vi "storeADCMixedToArray-wang-test2not simplified.vi"(0 "String":string) -> (18 "Graph Data":T1)   [LabVIEW 2014]
uses:
  main/controls/Graph Data.ctl
  <vilib>/Utility/miscctls.llb/LVAnnotationListTypeDef.ctl
  <vilib>/Utility/miscctls.llb/LVCursorListTypeDef.ctl
  main/global/Global ADCarray.vi
panel:
  out "header string":string
  in  "counter 2":i32
  out "Waveform":waveform(dbl)
  out "Graph":waveform(i32)[](graph)
  out "Numeric 2":i32
  out "Numeric":i32
  out "CH7":i32[](array[numeric])
  out "CH6":i32[](array[numeric])
  out "CH5":i32[](array[numeric])
  out "CH4":i32[](array[numeric])
  out "CH3":i32[](array[numeric])
  out "CH2":i32[](array[numeric])
  out "CH1":i32[](array[numeric])
  out "CH0":i32[](array[numeric])
  out "TotalTrigger":i32
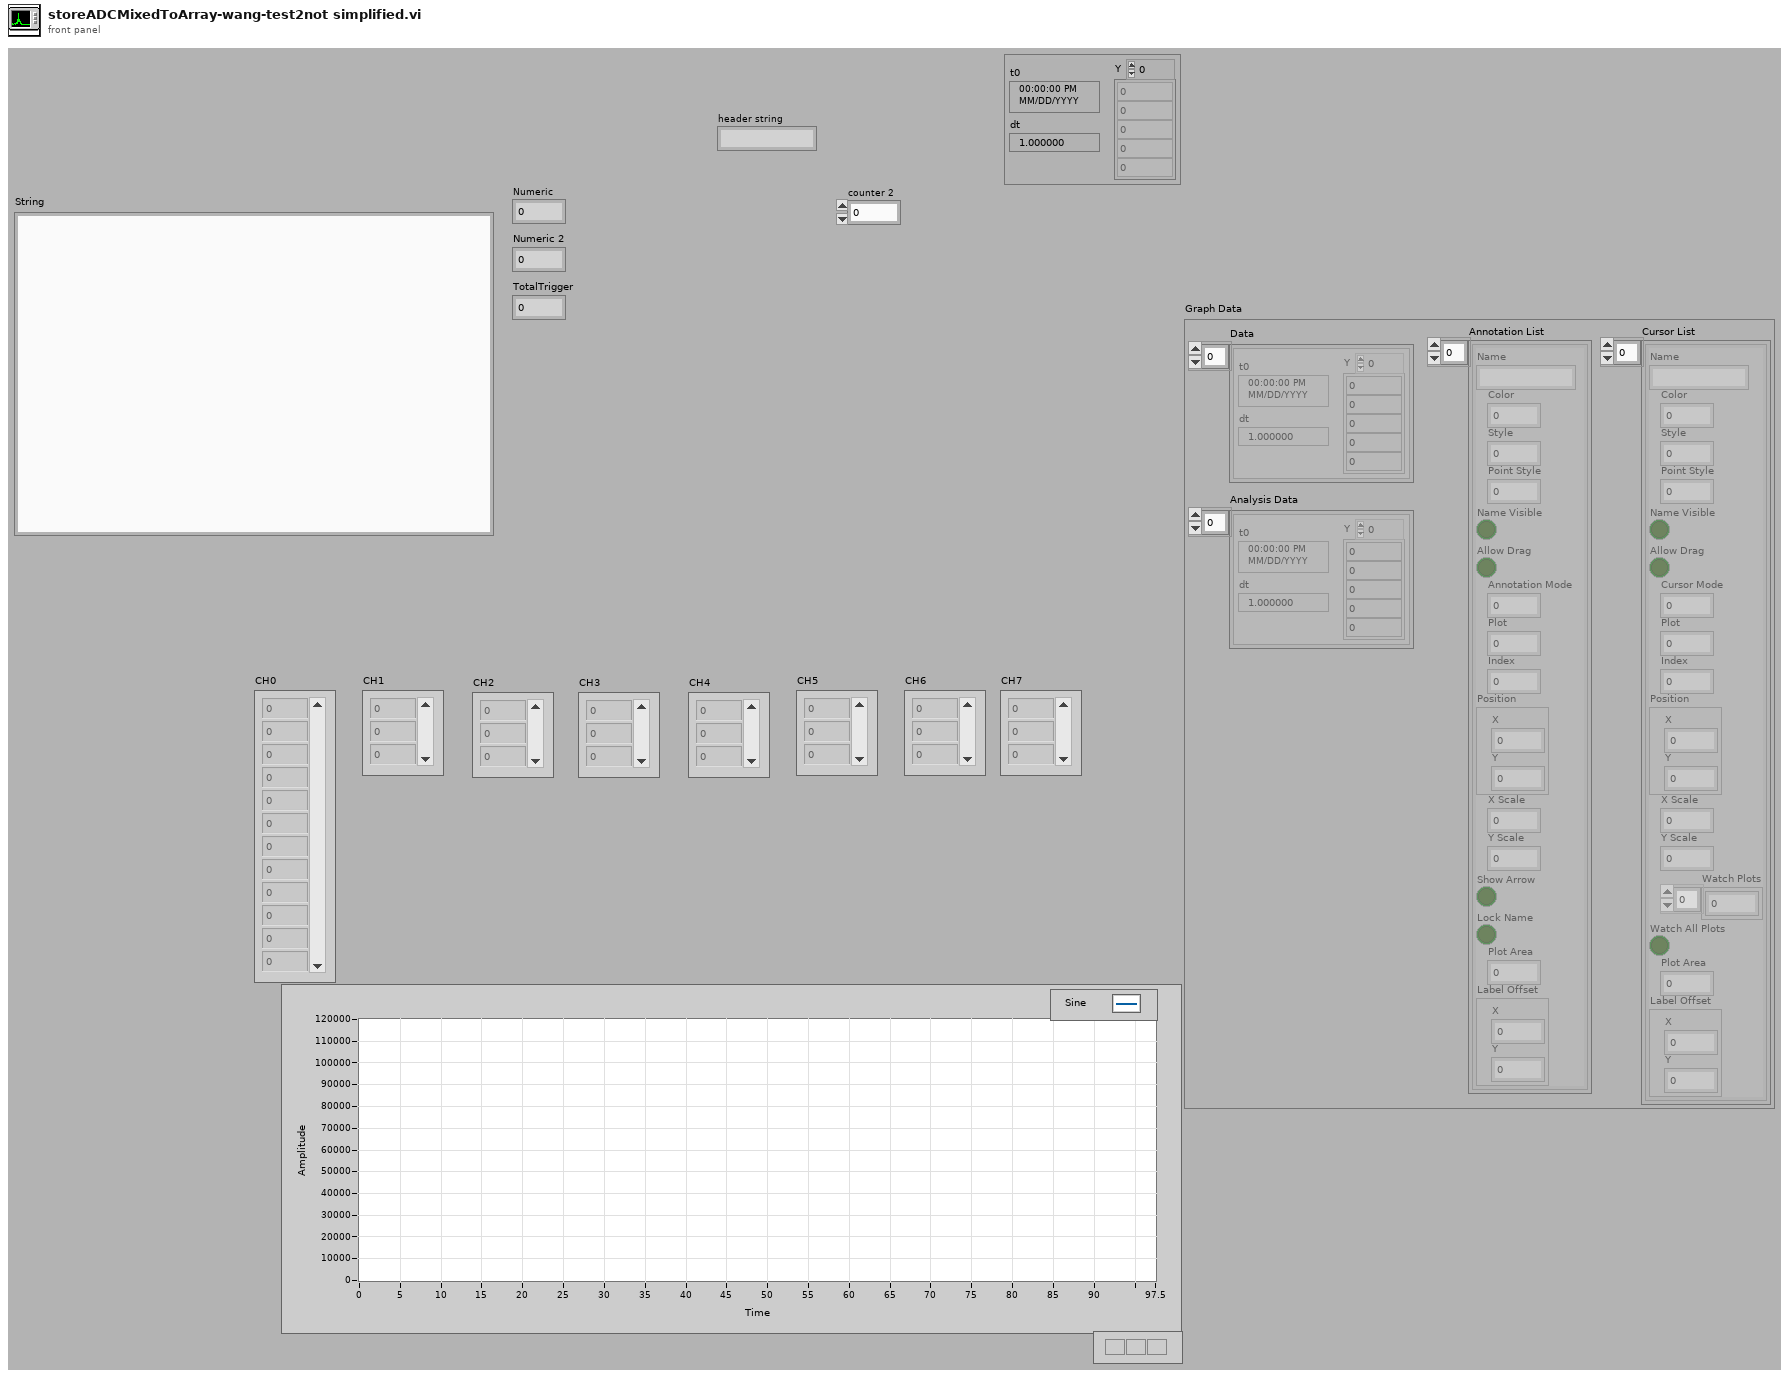
[diagram p1: front panel]
types:
  T1 = typedef "Graph Data.ctl" = cluster{"Data":waveform(dbl)[], "Annotation List":T2, "Cursor List":T3, "Analysis Data":waveform(dbl)[]}
  T2 = typedef "LVAnnotationListTypeDef.ctl" = cluster{"Name":string, "Color":u32, "Style":u8, "Point Style":u8, "Name Visible":bool, "Allow Drag":bool, "Annotation Mode":u32, "Plot":i32, "Index":i32, "Position":cluster{"X":dbl, "Y":dbl}, "X Scale":u32, "Y Scale":u32, "Show Arrow":bool, "Lock Name":bool, "Plot Area":i32, "Label Offset":cluster{"X":dbl, "Y":dbl}}[]
  T3 = typedef "LVCursorListTypeDef.ctl" = cluster{"Name":string, "Color":u32, "Style":u8, "Point Style":u8, "Name Visible":bool, "Allow Drag":bool, "Cursor Mode":u32, "Plot":i32, "Index":i32, "Position":cluster{"X":dbl, "Y":dbl}, "X Scale":u32, "Y Scale":u32, "Watch Plots":i32[], "Watch All Plots":bool, "Plot Area":i32, "Label Offset":cluster{"X":dbl, "Y":dbl}}[]
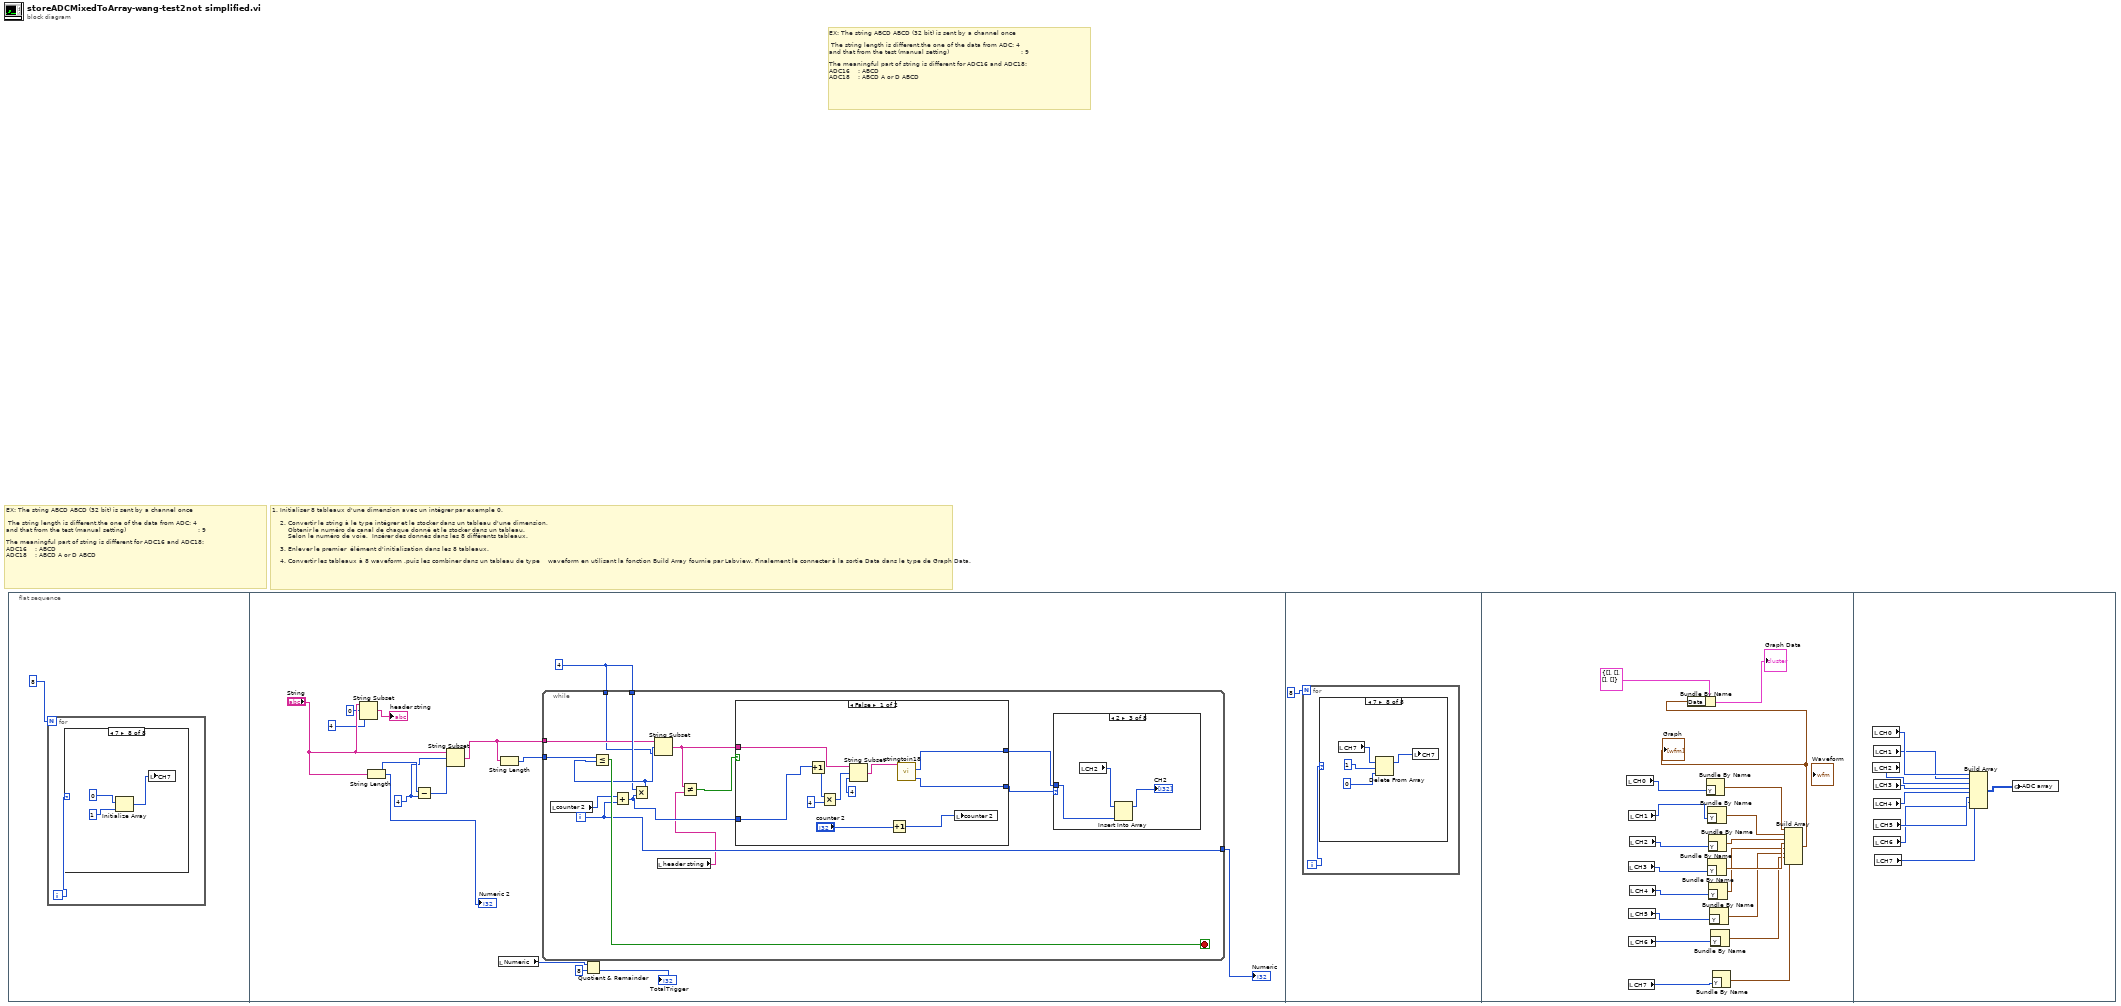
[diagram p0: block diagram]
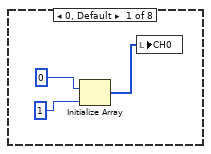
[diagram p2: hidden frame]
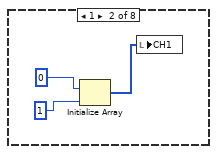
[diagram p3: hidden frame]
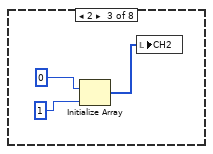
[diagram p4: hidden frame]
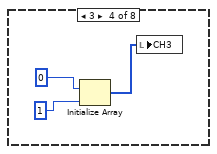
[diagram p5: hidden frame]
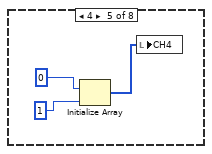
[diagram p6: hidden frame]
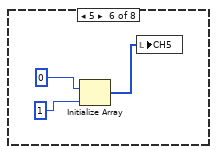
[diagram p7: hidden frame]
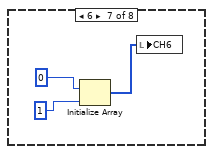
[diagram p8: hidden frame]
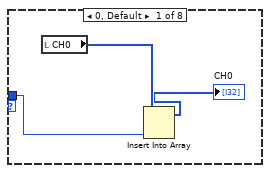
[diagram p9: hidden frame]
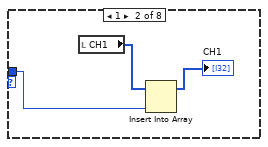
[diagram p10: hidden frame]
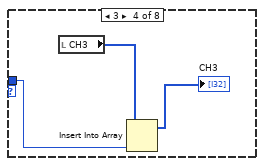
[diagram p11: hidden frame]
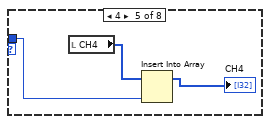
[diagram p12: hidden frame]
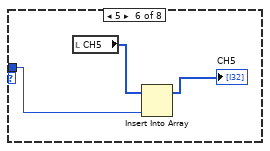
[diagram p13: hidden frame]
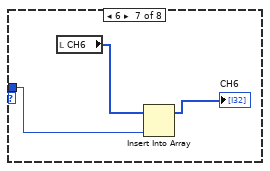
[diagram p14: hidden frame]
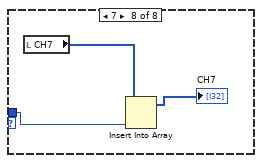
[diagram p15: hidden frame]
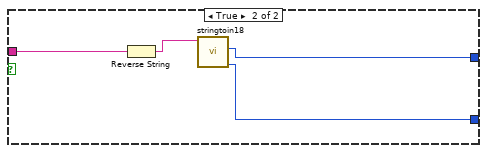
[diagram p16: hidden frame]
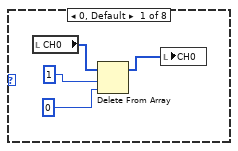
[diagram p17: hidden frame]
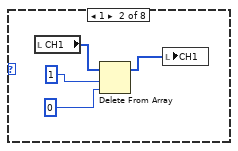
[diagram p18: hidden frame]
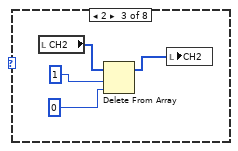
[diagram p19: hidden frame]
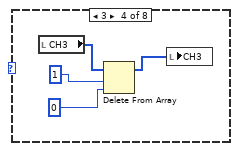
[diagram p20: hidden frame]
diagram:
  # "1. Initialiser 8 tableaux d'une dimension avec un intégrer par exemple 0.\n\n    2.\tConvertir le string à le type intégrer et le stocker dans un tableau d'une dimension,\n        Obtenir le numéro de canal de chaque donné et le stocker dans un tableau.  \n        Selon le numéro de voie,  Insérer des donnés dans les 8 différents tableaux.\n\n    3. Enlever le premier  élément d'initialisation dans les 8 tableaux.\n\n    4. Convertir les tableaux à 8 waveform ,puis les combiner dans un tableau de type    waveform en utilisant la fonction Build Array fournie par Labview. Finalement le connecter à la sortie Data dans le type de Graph Data."
  # "EX: The string ABCD ABCD (32 bit) is sent by a channel once                \n\n The string length is different,the one of the data from ADC: 4\nand that from the test (manual setting)                                    : 9\n\nThe meaningful part of string is different for ADC16 and ADC18:\nADC16    : ABCD                          \nADC18    : ABCD A or D ABCD"
  # "EX: The string ABCD ABCD (32 bit) is sent by a channel once                \n\n The string length is different,the one of the data from ADC: 4\nand that from the test (manual setting)                                    : 9\n\nThe meaningful part of string is different for ADC16 and ADC18:\nADC16    : ABCD                          \nADC18    : ABCD A or D ABCD"
  n1 = flat-sequence {
    frame #0 {
      n2 = for {
        N: 8 -> [_]
        i -> [w2]
        n3 = case shown="7" w2 {
          frame 0, Default {
            n4 = Initialize Array(0, 1) -> (w3:i32[])
            n5 = local write "CH0"(w3) -> ()
          }
          frame 1 {
            n6 = Initialize Array(0, 1) -> (w6:i32[])
            n7 = local write "CH1"(w6) -> ()
          }
          frame 2 {
            n8 = Initialize Array(0, 1) -> (w9:i32[])
            n9 = local write "CH2"(w9) -> ()
          }
          frame 3 {
            n10 = Initialize Array(0, 1) -> (w12:i32[])
            n11 = local write "CH3"(w12) -> ()
          }
          frame 4 {
            n12 = Initialize Array(0, 1) -> (w15:i32[])
            n13 = local write "CH4"(w15) -> ()
          }
          frame 5 {
            n14 = Initialize Array(0, 1) -> (w18:i32[])
            n15 = local write "CH5"(w18) -> ()
          }
          frame 6 {
            n16 = Initialize Array(0, 1) -> (w21:i32[])
            n17 = local write "CH6"(w21) -> ()
          }
          frame 7 {
            n18 = Initialize Array(0, 1) -> (w24:i32[])
            n19 = local write "CH7"(w24) -> ()
          }
        }
      }
    }
    frame #1 {
      w32 = 4
      w38 = 4
      n20 = String Subset(string="String", offset (0)=0, length (rest)=4 ("length (rest)")) -> (substring=→"header string":string)
      n21 = String Length(string="String") -> (length=w40:i32)
      "Numeric 2" <- w40
      n22 = Subtract(x=w40, y=w38) -> (x-y=w39:i32)
      n23 = String Subset(string="String", offset (0)=w38, length (rest)=w39) -> (substring=w34:string)
      n24 = local read "Numeric"() -> (w35:i32)
      n25 = String Length(string=w34) -> (length=w33:i32)
      n26 = while {
        tunnel: [w52] -> w31
        tunnel: w32 -> [w49]
        tunnel: w34 -> [w48]
        tunnel: w33 -> [w47]
        tunnel: w32 -> [w46]
        i -> [w52]
        stop <- w53 stop-if-true
        n27 = local read "counter 2"() -> (w42:i32)
        n28 = Add(x=w42, y=w52) -> (x+y=w50:i32)
        n29 = Multiply(x=w49, y=w50) -> (x*y=w51:i32)
        n30 = Less Or Equal?(x=w47, y=w51) -> (x <= y?=w53:bool)
        n31 = String Subset(string=w48, offset (0)=w51, length (rest)=w46) -> (substring=w54:string)
        n32 = local read "header string"() -> (w41:string)
        n33 = Not Equal?(x=w54, y=w41) -> (x != y?=w43:bool)
        n34 = case shown="False" w43 {
          tunnel: [w88 w93] -> w44
          tunnel: [w87 w92] -> w45
          tunnel: w54 -> [w85 w90]
          tunnel: w50 -> [w82 _]
          frame False {
            n35 = Increment(x=w82) -> (x+1=w81:i32)
            n36 = Multiply(x=w81, y=4) -> (x*y=w86:i32)
            n37 = String Subset(string=w85, offset (0)=w86, length (rest)=4) -> (substring=w79:string)
            n38 = Increment(x="counter 2") -> (x+1=w80:i32)
            n39 = call "stringtoin18.vi"("input_string"=w79) -> ("channel"=w87:u8, "outputComplemented_int"=w88:i32)  [unwired: 7 in, 2 out]
            n40 = local write "counter 2"(w80) -> ()
          }
          frame True {
            n41 = Reverse String(1:w90) -> (0:w91:string)
            n42 = call "stringtoin18.vi"("input_string"=w91) -> ("channel"=w92:u8, "outputComplemented_int"=w93:i32)  [unwired: 7 in, 2 out]
          }
        }
        n43 = case shown="2" w45 {
          tunnel: w44 -> [w55 w58 w61 w64 w67 w70 w73 w76]
          frame 0, Default {
            n44 = local read "CH0"() -> (w57:i32[])
            n45 = Insert Into Array(array=w57, new element=w55) -> (→"CH0":i32[])  [unwired: 1 in]
          }
          frame 1 {
            n46 = local read "CH1"() -> (w60:i32[])
            n47 = Insert Into Array(array=w60, new element=w58) -> (→"CH1":i32[])  [unwired: 1 in]
          }
          frame 2 {
            n48 = local read "CH2"() -> (w63:i32[])
            n49 = Insert Into Array(array=w63, new element=w61) -> (→"CH2":i32[])  [unwired: 1 in]
          }
          frame 3 {
            n50 = local read "CH3"() -> (w66:i32[])
            n51 = Insert Into Array(array=w66, new element=w64) -> (→"CH3":i32[])  [unwired: 1 in]
          }
          frame 4 {
            n52 = local read "CH4"() -> (w69:i32[])
            n53 = Insert Into Array(array=w69, new element=w67) -> (→"CH4":i32[])  [unwired: 1 in]
          }
          frame 5 {
            n54 = local read "CH5"() -> (w72:i32[])
            n55 = Insert Into Array(array=w72, new element=w70) -> (→"CH5":i32[])  [unwired: 1 in]
          }
          frame 6 {
            n56 = local read "CH6"() -> (w75:i32[])
            n57 = Insert Into Array(array=w75, new element=w73) -> (→"CH6":i32[])  [unwired: 1 in]
          }
          frame 7 {
            n58 = local read "CH7"() -> (w77:i32[])
            n59 = Insert Into Array(array=w77, new element=w76) -> (→"CH7":i32[])  [unwired: 1 in]
          }
        }
      }
      "Numeric" <- w31
      n60 = Quotient & Remainder(x=w35, y=8) -> (floor(x/y)=→"TotalTrigger":i32)  [unwired: 1 out]
    }
    frame #2 {
      n61 = for {
        N: 8 -> [_]
        i -> [w95]
        n62 = case shown="7" w95 {
          frame 0, Default {
            n63 = local read "CH0"() -> (w99:i32[])
            n64 = Delete From Array(array=w99, length=1, index=0) -> (array with subset deleted=w96:i32[])  [unwired: 1 out]
            n65 = local write "CH0"(w96) -> ()
          }
          frame 1 {
            n66 = local read "CH1"() -> (w103:i32[])
            n67 = Delete From Array(array=w103, length=1, index=0) -> (array with subset deleted=w100:i32[])  [unwired: 1 out]
            n68 = local write "CH1"(w100) -> ()
          }
          frame 2 {
            n69 = local read "CH2"() -> (w107:i32[])
            n70 = Delete From Array(array=w107, length=1, index=0) -> (array with subset deleted=w104:i32[])  [unwired: 1 out]
            n71 = local write "CH2"(w104) -> ()
          }
          frame 3 {
            n72 = local read "CH3"() -> (w111:i32[])
            n73 = Delete From Array(array=w111, length=1, index=0) -> (array with subset deleted=w108:i32[])  [unwired: 1 out]
            n74 = local write "CH3"(w108) -> ()
          }
          frame 4 {
            n75 = local read "CH4"() -> (w115:i32[])
            n76 = Delete From Array(array=w115, length=1, index=0) -> (array with subset deleted=w112:i32[])  [unwired: 1 out]
            n77 = local write "CH4"(w112) -> ()
          }
          frame 5 {
            n78 = local read "CH5"() -> (w119:i32[])
            n79 = Delete From Array(array=w119, length=1, index=0) -> (array with subset deleted=w116:i32[])  [unwired: 1 out]
            n80 = local write "CH5"(w116) -> ()
          }
          frame 6 {
            n81 = local read "CH6"() -> (w123:i32[])
            n82 = Delete From Array(array=w123, length=1, index=0) -> (array with subset deleted=w120:i32[])  [unwired: 1 out]
            n83 = local write "CH6"(w120) -> ()
          }
          frame 7 {
            n84 = local read "CH7"() -> (w127:i32[])
            n85 = Delete From Array(array=w127, length=1, index=0) -> (array with subset deleted=w124:i32[])  [unwired: 1 out]
            n86 = local write "CH7"(w124) -> ()
          }
        }
      }
    }
    frame #3 {
      n87 = local read "CH0"() -> (w146:i32[])
      n88 = local read "CH3"() -> (w138:i32[])
      n89 = local read "CH7"() -> (w142:i32[])
      n90 = local read "CH1"() -> (w144:i32[])
      n91 = local read "CH5"() -> (w140:i32[])
      n92 = local read "CH6"() -> (w141:i32[])
      n93 = local read "CH2"() -> (w137:i32[])
      n94 = local read "CH4"() -> (w139:i32[])
      n95 = Bundle By Name("Y"=w146) -> (w145:waveform(i32))  [unwired: 1 in]
      n96 = Bundle By Name("Y"=w144) -> (w143:waveform(i32))  [unwired: 1 in]
      n97 = Bundle By Name("Y"=w138) -> (w135:waveform(i32))  [unwired: 1 in]
      n98 = Bundle By Name("Y"=w137) -> (w136:waveform(i32))  [unwired: 1 in]
      n99 = Bundle By Name("Y"=w139) -> (w131:waveform(i32))  [unwired: 1 in]
      n100 = Bundle By Name("Y"=w140) -> (w134:waveform(i32))  [unwired: 1 in]
      n101 = Bundle By Name("Y"=w141) -> (w133:waveform(i32))  [unwired: 1 in]
      n102 = Bundle By Name("Y"=w142) -> (w132:waveform(i32))  [unwired: 1 in]
      n103 = Build Array(w145, w143, w136, w135, w131, w134, w133, w132) -> (w130:waveform(i32)[])
      "Graph" <- w130
      n104 = Bundle By Name(cluster=T1 {"Data"=[], "Annotation List"=[], "Cursor List"=[], "Analysis Data"=[]} ("Graph Data"), "Data"=w130) -> (→"Graph Data":T1)
    }
    frame #4 {
      n105 = local read "CH0"() -> (w155:i32[])
      n106 = local read "CH2"() -> (w153:i32[])
      n107 = local read "CH1"() -> (w154:i32[])
      n108 = local read "CH3"() -> (w152:i32[])
      n109 = local read "CH4"() -> (w151:i32[])
      n110 = local read "CH5"() -> (w150:i32[])
      n111 = local read "CH6"() -> (w149:i32[])
      n112 = local read "CH7"() -> (w148:i32[])
      n113 = Build Array(w155, w154, w153, w152, w151, w150, w149, w148) -> (w147:i32[][])
      n114 = global write "Global ADCarray.vi" "ADC array"(w147) -> ()
    }
  }
